vi "PowerStatusChanged.vi"(7 "ControlQueue":refnum<queue>, 8 "entrée d'erreur (pas d'erreur)":errorcluster, 9 "PowerStatus":bool, 10 "PowerStatusChanged":bool, 11 "DAQmxTaskContainer en entrée":refnum<class "DAQmxTaskContainer.lvclass">) -> (0 "sortie d'erreur":errorcluster, 3 "DAQmxTaskContainer en sortie":refnum<class "DAQmxTaskContainer.lvclass">)   [LabVIEW 2015, in "DAQmxTaskContainer.lvclass"]
uses:
  DAQmxTaskContainer.lvclass
  dependecies/ControlsVIs/Clusters-def/ProtypeCommand-DAQmxReply.ctl
  dependecies/ControlsVIs/Clusters-def/SERVER-Commands.ctl
  dependecies/ControlsVIs/Clusters-def/Standard Command.ctl
  DAQmxTaskContainer.lvclass/DAQmxTaskContainer.ctl
  Control/Control-Server/Control-Server.lvclass
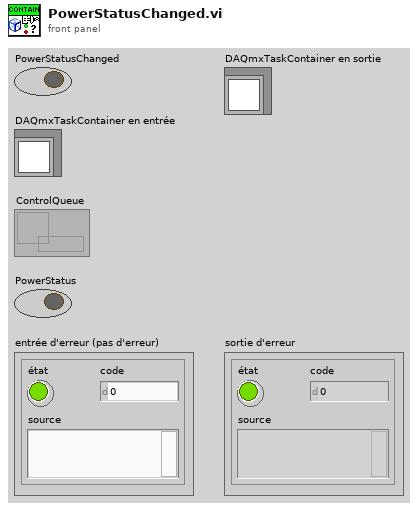
[diagram p1: front panel]
types:
  T1 = typedef "Standard Command.ctl" = cluster{"command":string, "data":variant}
  T2 = typedef "Control-Server.lvclass/SERVER-Commands.ctl" = string
  T3 = typedef "ProtypeCommand-DAQmxReply.ctl" = cluster{"On/Off":bool, "error out":errorcluster}
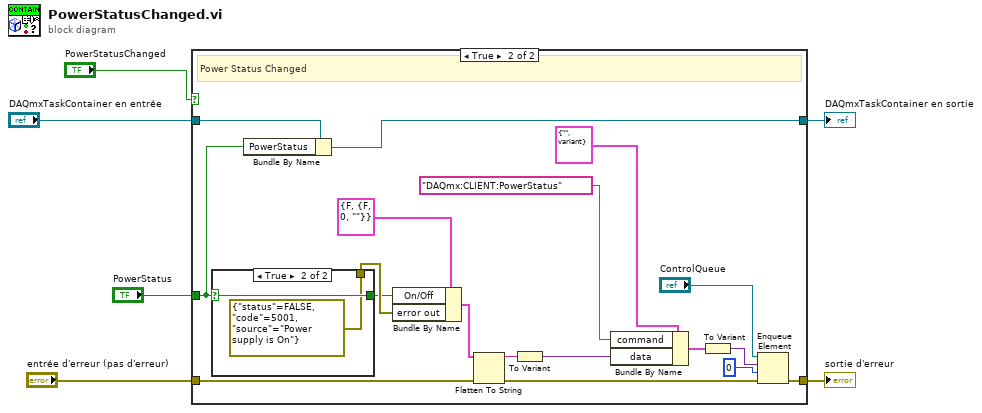
[diagram p0: block diagram]
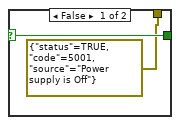
[diagram p3: hidden frame]
diagram:
  n1 = case shown="True" "PowerStatusChanged" {
    tunnel: "DAQmxTaskContainer en entrée" -> [w8 w16]
    tunnel: [w8 w13] -> w6
    tunnel: "entrée d'erreur (pas d'erreur)" -> [w7 w19]
    tunnel: [w7 w17] -> w1
    tunnel: "PowerStatus" -> [_ w10]
    frame False {
    }
    frame True {
      # "Power Status Changed"
      n2 = case shown="True" w10 {
        selector: w10 -> [w28 w30]
        tunnel: [w28 w30] -> w20
        tunnel: [errorcluster {"status"=TRUE, "code"=5001, "source"="Power supply is Off"} ("error out") errorcluster {"status"=FALSE, "code"=5001, "source"="Power supply is On"} ("error out")] -> w21
        frame False {
        }
        frame True {
        }
      }
      n3 = Bundle By Name(cluster=w16, "PowerStatus"=w10) -> (w13:refnum<class "DAQmxTaskContainer.lvclass">)
      n4 = Bundle By Name(cluster=T3 {"On/Off"=FALSE, "error out"={"status"=FALSE, "code"=0, "source"=""}} ("output cluster"), "On/Off"=w20, "error out"=w21) -> (w25:T3)
      n5 = Flatten To String(anything=w25, error in (no error)=w19) -> (data string=w23:string, error out=w18:errorcluster)  [unwired: 2 in, 1 out]
      n6 = To Variant(anything=w23) -> (Variant=w24:variant)
      n7 = Bundle By Name(cluster=T1 {"command"="", "data"=variant} ("input cluster"), "command"=T2 "DAQmx:CLIENT:PowerStatus" ("Commands"), "data"=w24) -> (w15:T1)
      n8 = To Variant(anything=w15) -> (Variant=w14:variant)
      n9 = Enqueue Element(queue="ControlQueue", element=w14, timeout in ms (-1)=0 ("timeout en ms (-1)"), error in (no error)=w18) -> (error out=w17:errorcluster)  [unwired: 2 out]
    }
  }
  "DAQmxTaskContainer en sortie" <- w6
  "sortie d'erreur" <- w1
